vi "Read Data From BMP File.vi"(8 "错误输入":errorcluster, 11 "文件（使用对话框）":path) -> (0 "错误输出":errorcluster, 3 "数据":string)   [LabVIEW 2012, in "Picture Box Tools.lvlib" / "BMP File.lvlib"]
uses:
  BMP File.lvlib
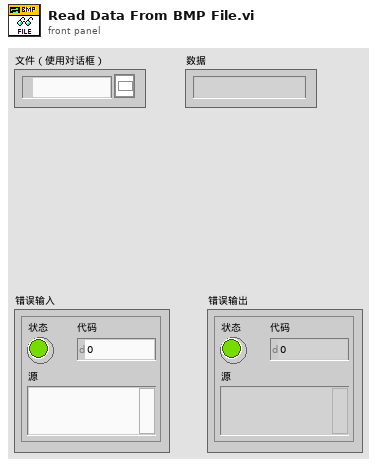
[diagram p1: front panel]
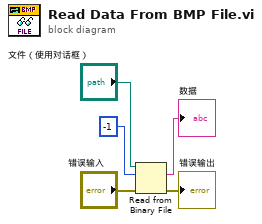
[diagram p0: block diagram]
diagram:
  n1 = Read from Binary File(8:"错误输入", 10:-1 ("总数(1)"), 11:"文件（使用对话框）") -> (0:→"错误输出":errorcluster, 2:→"数据":string)  [unwired: 3 in, 2 out]
